vi "Write Input B.vi"(8 "error in (no error)":errorcluster, 10 "Abs_Time.lvclass":refnum<class "Abs_Time.lvclass">, 11 "Subtract_Time in":refnum<class "Subtract_Time-Time.lvclass">) -> (0 "error out":errorcluster, 3 "Subtract_Time out":refnum<class "Subtract_Time-Time.lvclass">)   [LabVIEW 2021, in "Subtract_Time-Time.lvclass"]
uses:
  Subtract_Time-Time.lvclass
  Abs_Types/Time/Abs_Time.lvclass
  Subtract_Time-Time.lvclass/Subtract_Time-Time.ctl
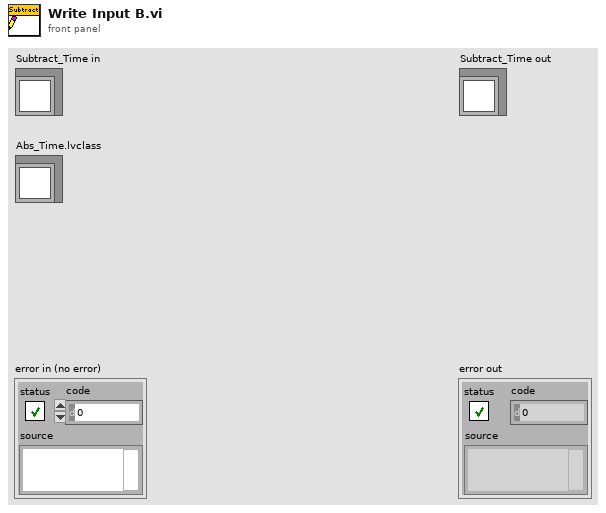
[diagram p1: front panel]
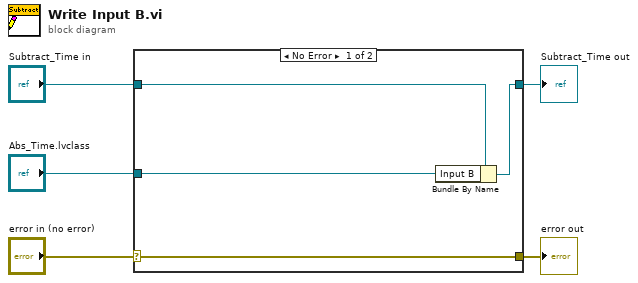
[diagram p0: block diagram]
diagram:
  n1 = case shown="No Error" "error in (no error)" {
    selector: "error in (no error)" -> [w9 w10]
    tunnel: [w9 w10] -> w4
    tunnel: [w7 w11] -> w2
    tunnel: "Subtract_Time in" -> [w8 w11]
    tunnel: "Abs_Time.lvclass" -> [w6 _]
    frame No Error {
      n2 = Bundle By Name(cluster=w8, "Input B"=w6) -> (w7:refnum<class "Subtract_Time-Time.lvclass">)
    }
    frame Error {
    }
  }
  "error out" <- w4
  "Subtract_Time out" <- w2
